vi "SubConfocal_GetDiskSpinningSpeed.vi"(8 "Error In":errorcluster, 11 "Confocal line (VISA IN)":refnum<visa-resource-name>="COM1") -> (0 "Error out":errorcluster, 3 "VISA OUT":refnum<visa-resource-name>, 5 "Actual Disk speed (rpm)":string="0")   [LabVIEW 2015]
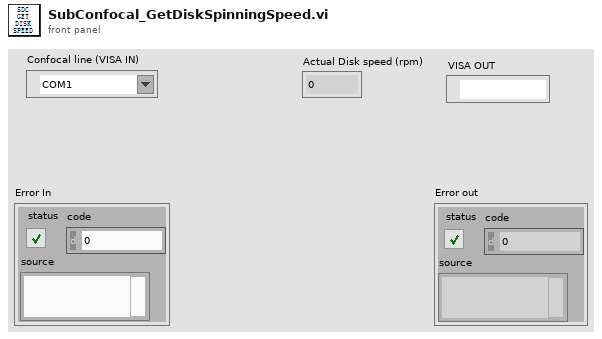
[diagram p1: front panel]
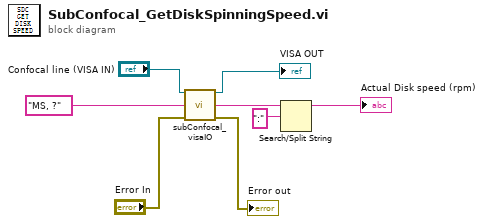
[diagram p0: block diagram]
diagram:
  n1 = call "subConfocal_visaIO.vi"("VISA  IN"="Confocal line (VISA IN)", "Command (to ctlr)"="MS, ?", "error in"="Error In") -> ("VISA OUT"=→"VISA OUT":refnum<visa-resource-name>, "Raw Response"=w8:string, "error out"=→"Error out":errorcluster)  [unwired: 8 in, 2 out]
  n2 = Search/Split String(string=w8, search string/char (-)=":") -> (substring before match=→"Actual Disk speed (rpm)":string)  [unwired: 1 in, 2 out]
